vi "Cypher Lithography 2.0_Feng_MFP3D_Lucy.vi"(0 "Nodes on the line\n(  x      ,       y   )":dbl[][](array[numeric])=[[-5e-06, -5e-06], [5e-06, 5e-06]] min=-4.5e-05 max=4.5e-05 step=1e-09 format="%#_6pm", 1 "V":dbl[](array[numeric]), 2 "Litho Speed":dbl=5e-07 format="%#_6pm/s", 3 "Z SetPoint":dbl format="%#_6p", 4 "New nodes spacing":dbl=1e-06 format="%#_6pm", 5 "display wave":bool, 6 "Need interpolate new nodes?":bool, 7 "PID close":bool) -> ()   [LabVIEW 2016]
uses:
  Cypher XY LVDT Parameters_MFP3D_Lucy.vi
  <vilib>/Analysis/2dsp.llb/Resample (constant to constant,single -channel).vi
  <vilib>/Utility/file.llb/Write To Spreadsheet File (DBL).vi
  <vilib>/Analysis/NI_AALPro.lvlib
panel:
  out "size(s) 3":i32
  out "size(s) 2":i32[](array[numeric])
  out "size(s)":i32[](array[numeric])
  out "XY Graph":T1(graph)
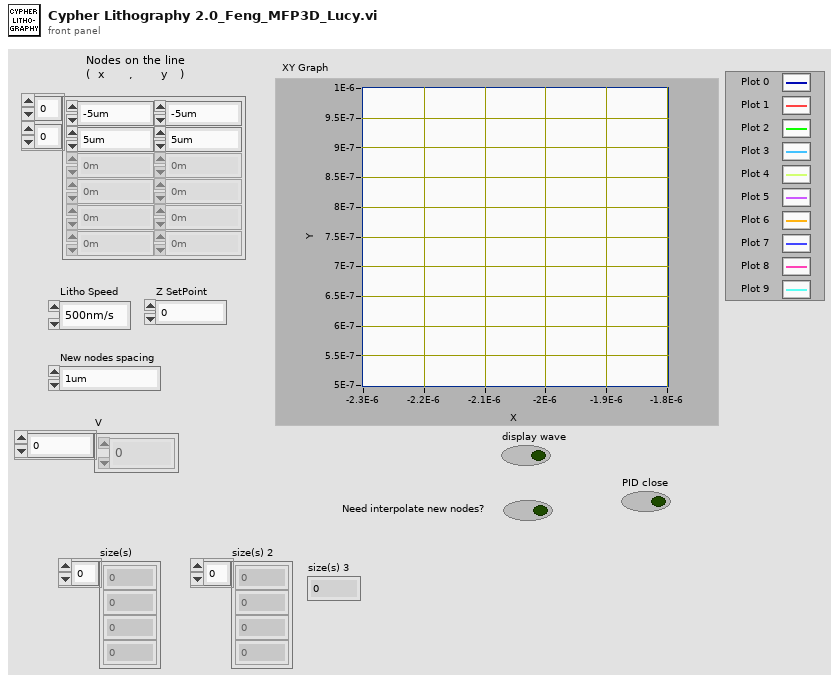
[diagram p1: front panel]
types:
  T1 = cluster{"Nodes on the line\n(  x      ,       y   )":dbl[], "Nodes on the line\n(  x      ,       y   )":dbl[]}[]
  T2 = cluster{"Interpolate result":dbl[], "Interpolate result":dbl[]}
  T3 = enum16{"open", "replace", "create", "open or create", "replace or create", "replace or create with confirmation"}
  T4 = cluster{"Nodes on the line\n(  x      ,       y   )":dbl[], "Nodes on the line\n(  x      ,       y   )":dbl[]}
  T5 = cluster{"Interpolate result":dbl[], "Interpolate result":dbl[]}[]
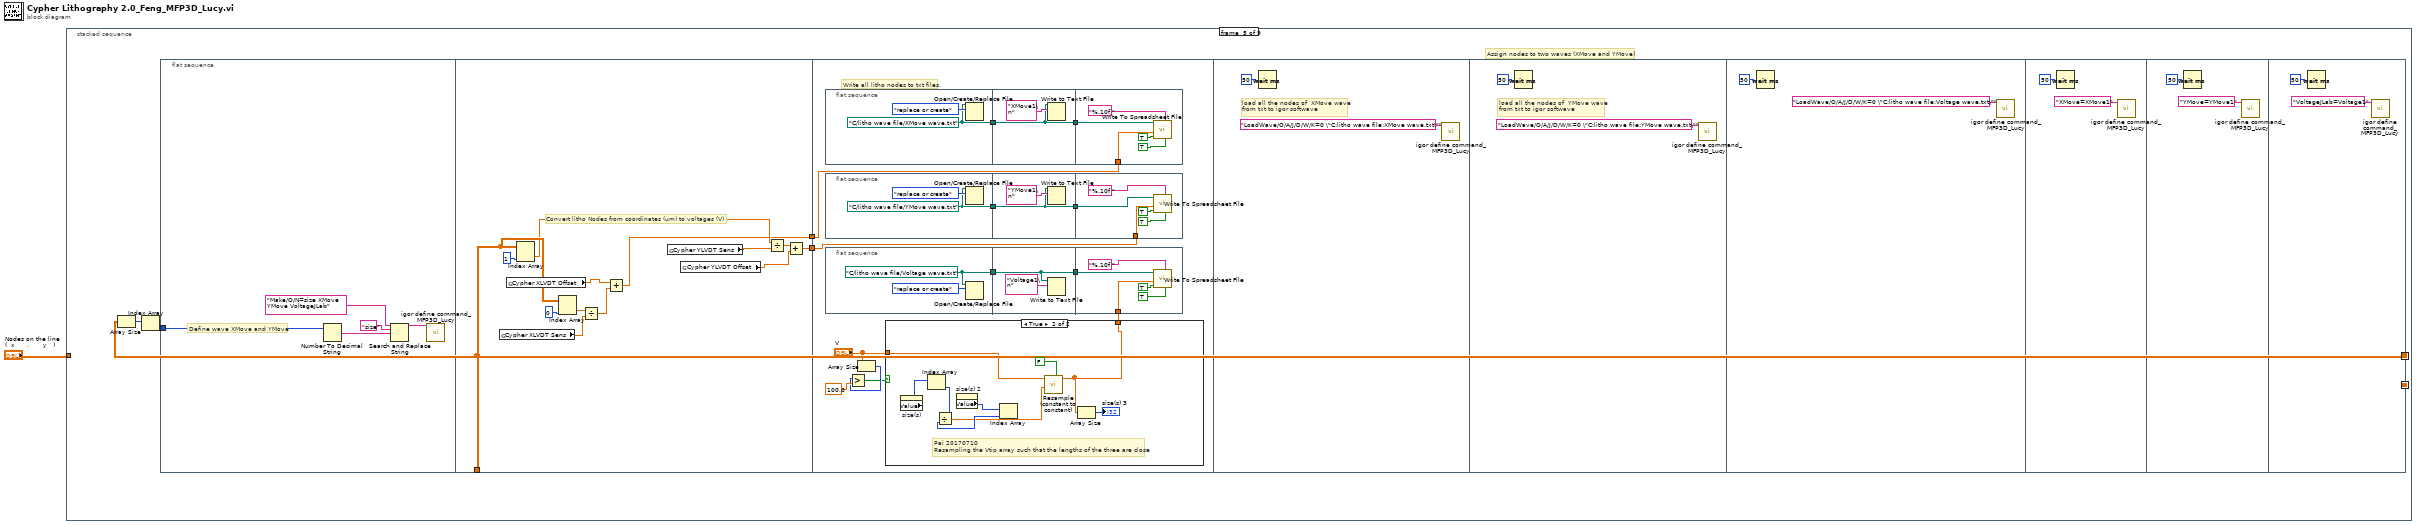
[diagram p0: block diagram]
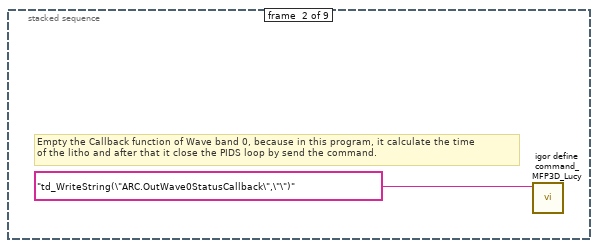
[diagram p3: hidden frame]
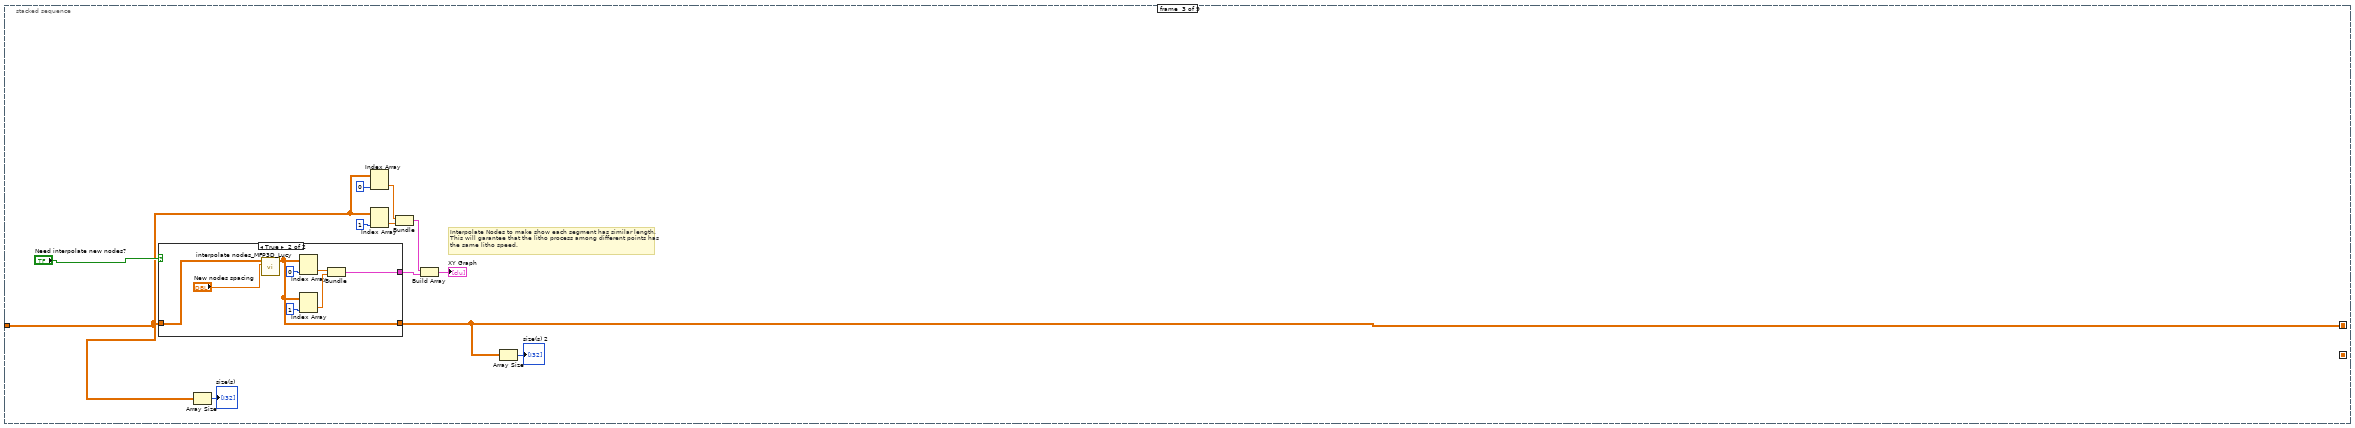
[diagram p4: hidden frame]
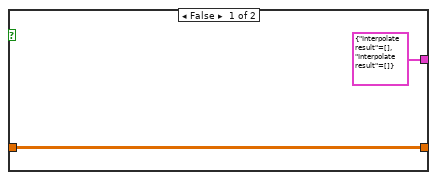
[diagram p5: hidden frame]
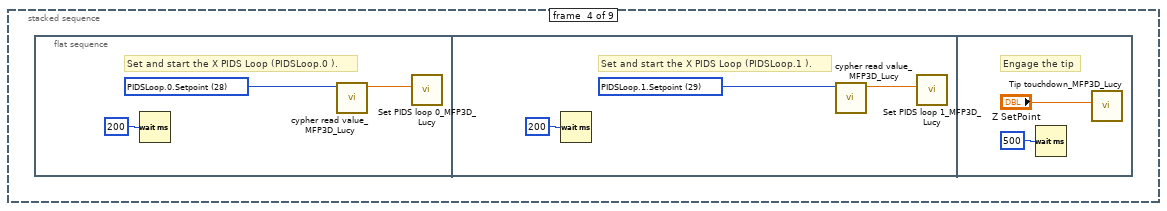
[diagram p6: hidden frame]
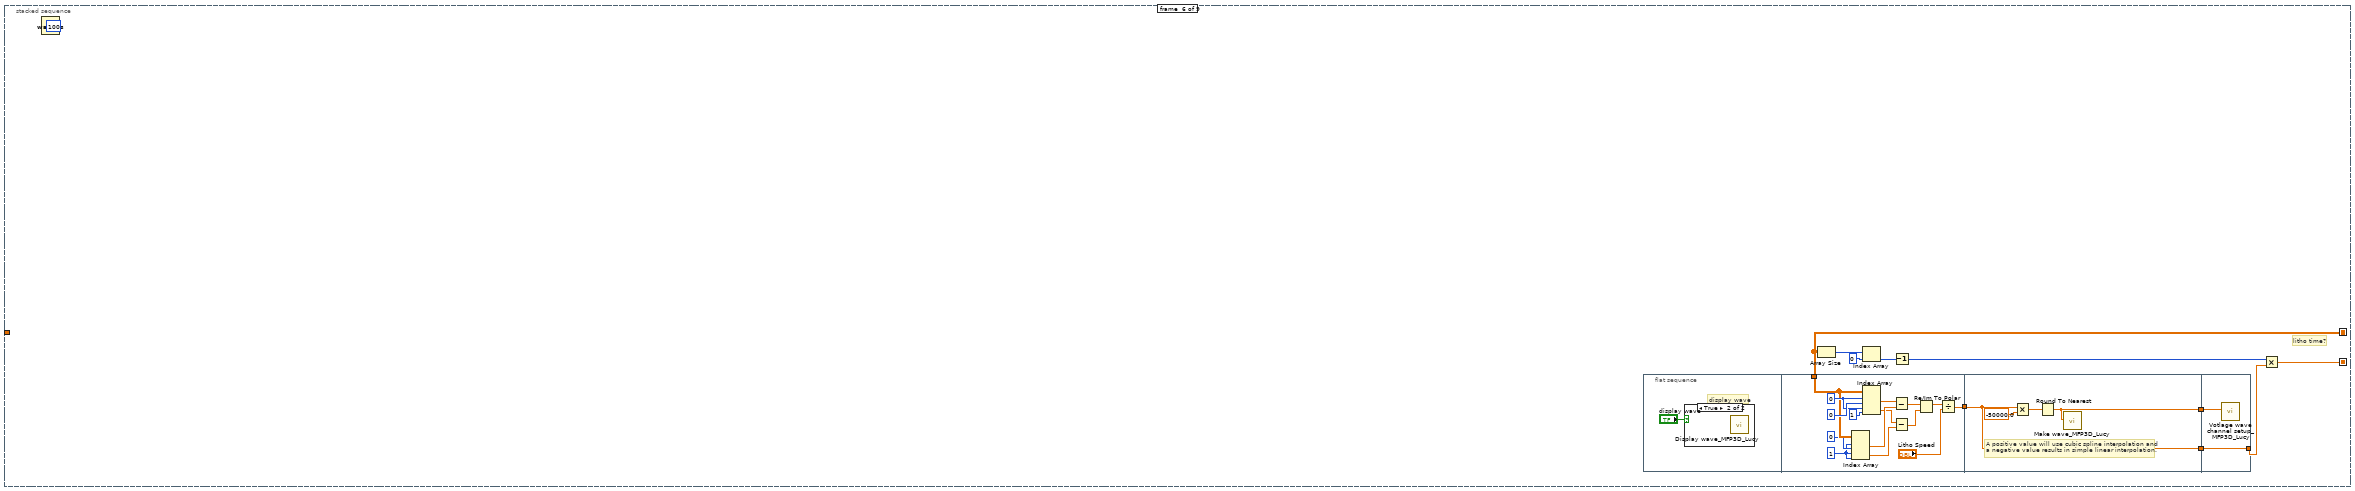
[diagram p8: hidden frame]
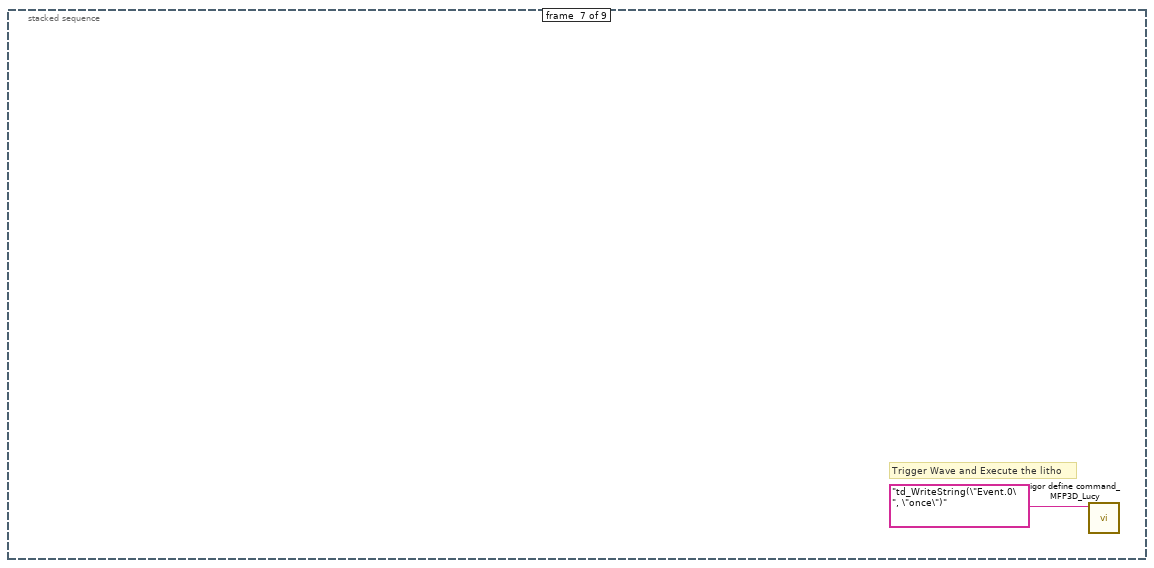
[diagram p10: hidden frame]
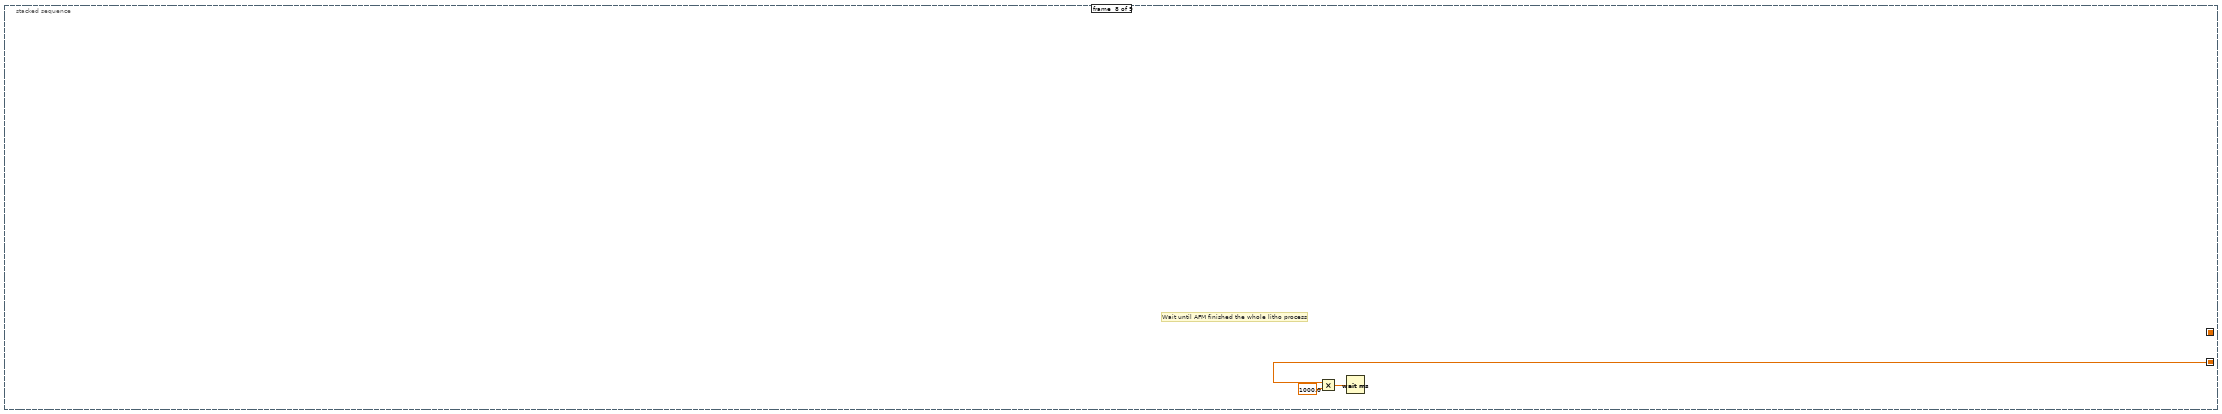
[diagram p11: hidden frame]
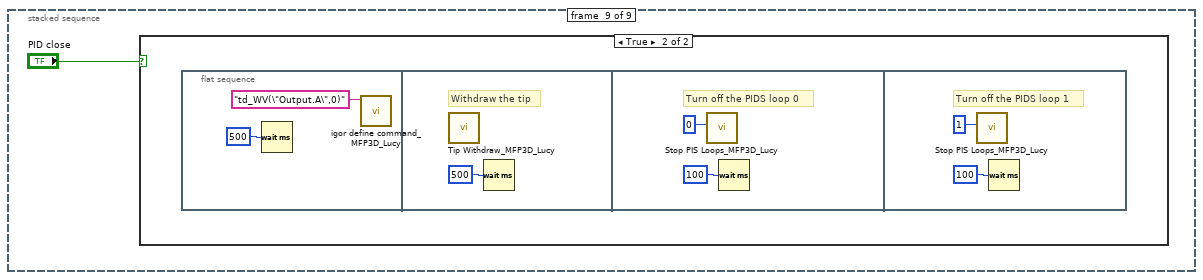
[diagram p12: hidden frame]
diagram:
  n1 = stacked-sequence {
    seq-local: [_ _ w3 _ _ _ _ _ _] -> [_ _ _ _ w34 w127 _ _ _]
    seq-local: [_ _ _ _ _ w123 _ _ _] -> [_ _ _ _ _ _ _ w154 _]
    tunnel: "Nodes on the line\n(  x      ,       y   )" -> [_ _ w6 _ _ _ _ _ _]
    frame #0 {
    }
    frame #1 {
      # "Empty the Callback function of Wave band 0, because in this program, it calculate the time \nof the litho and after that it close the PIDS loop by send the command."
      n2 = call "igor define command_MFP3D_Lucy.vi"("Command"="td_WriteString(\"ARC.OutWave0StatusCallback\",\"\")") -> ()  [unwired: 11 out]
    }
    frame #2 {
      # "Interpolate Nodes to make show each segment has similar length.\nThis will garantee that the litho process among different points has\nthe same litho speed."
      n3 = case shown="True" "Need interpolate new nodes?" {
        tunnel: w6 -> [w16 w17]
        tunnel: [T2 {"Interpolate result"=[], "Interpolate result"=[]} w20] -> w8
        tunnel: [w16 w19] -> w3
        frame False {
        }
        frame True {
          n4 = call "interpolate nodes_MFP3D_Lucy.vi"("Interpolate spacing"="New nodes spacing", "Nodes on the line\n(  x      ,       y   )"=w17) -> ("Interpolate result"=w19:dbl[][])  [unwired: 9 in]
          n5 = Index Array(array=w19, index (col)=0 ("disabled index (col)")) -> (element=w22:dbl[])  [unwired: 1 in]
          n6 = Index Array(array=w19, index (col)=1 ("disabled index (col)")) -> (element=w21:dbl[])  [unwired: 1 in]
          n7 = Bundle("Interpolate result"=w22, "Interpolate result"=w21) -> (w20:T2)  [unwired: 1 in]
        }
      }
      n8 = Array Size(array=w6) -> (size(s)=→"size(s)":i32[])
      n9 = Index Array(array=w6, index (col)=0 ("disabled index (col)")) -> (element=w13:dbl[])  [unwired: 1 in]
      n10 = Index Array(array=w6, index (col)=1 ("disabled index (col)")) -> (element=w11:dbl[])  [unwired: 1 in]
      n11 = Bundle("Nodes on the line\n(  x      ,       y   )"=w13, "Nodes on the line\n(  x      ,       y   )"=w11) -> (w10:T4)  [unwired: 1 in]
      n12 = Build Array(w10, w8) -> (→"XY Graph":T5)
      n13 = Array Size(array=w3) -> (size(s)=→"size(s) 2":i32[])
    }
    frame #3 {
      n14 = flat-sequence {
        frame #0 {
          w26 = u16 28 items=["XSensor", "YSensor", "ZSensor", "InA", "InB", "InFast", "In_Amplitude1", "In_Amplitude2", "In_Phase1", "In_Phase2", "PiezoX", "PiezoY", "PiezoZ", "OutA", "OutB", "OutC", "DDS_Frequency1", "DDS_Frequency2", "DDS_Amplitude1", "DDS_Amplitude2", "DDS_DCOffset", "Laser_Sum", "Laser_Difference", "Laser_Lateral", "XLVDT Sensitivity", "YLVDT Sensitivity", "XLVDT Offset", "YLVDT Offset", "PIDSLoop.0.Setpoint", "PIDSLoop.1.Setpoint"] ("Input")
          # "Set and start the X PIDS Loop (PIDSLoop.0 )."
          n15 = Wait (ms)(milliseconds to wait=u32 200) -> ()  [unwired: 1 out]
          n16 = call "cypher read value_MFP3D_Lucy.vi"("Input"=w26) -> ("Result"=w27:dbl)  [unwired: 10 in]
          n17 = call "Set PIDS loop 0_MFP3D_Lucy.vi"("X  Setpoint"=w27) -> ()  [unwired: 11 in]
        }
        frame #1 {
          w29 = u16 29 items=["XSensor", "YSensor", "ZSensor", "InA", "InB", "InFast", "In_Amplitude1", "In_Amplitude2", "In_Phase1", "In_Phase2", "PiezoX", "PiezoY", "PiezoZ", "OutA", "OutB", "OutC", "DDS_Frequency1", "DDS_Frequency2", "DDS_Amplitude1", "DDS_Amplitude2", "DDS_DCOffset", "Laser_Sum", "Laser_Difference", "Laser_Lateral", "XLVDT Sensitivity", "YLVDT Sensitivity", "XLVDT Offset", "YLVDT Offset", "PIDSLoop.0.Setpoint", "PIDSLoop.1.Setpoint"] ("Input")
          # "Set and start the X PIDS Loop (PIDSLoop.1 )."
          n18 = Wait (ms)(milliseconds to wait=u32 200) -> ()  [unwired: 1 out]
          n19 = call "cypher read value_MFP3D_Lucy.vi"("Input"=w29) -> ("Result"=w30:dbl)  [unwired: 10 in]
          n20 = call "Set PIDS loop 1_MFP3D_Lucy.vi"("Y Setpoint"=w30) -> ()  [unwired: 11 in]
        }
        frame #2 {
          # "Engage the tip"
          n21 = Wait (ms)(milliseconds to wait=u32 500) -> ()  [unwired: 1 out]
          n22 = call "Tip touchdown_MFP3D_Lucy.vi"("Z SetPoint"="Z SetPoint") -> ()  [unwired: 11 out]
        }
      }
    }
    frame #4 {
      # "Assign nodes to two waves (XMove and YMove)"
      n23 = Array Size(array=w34) -> (size(s)=w35:i32[])
      n24 = Index Array(array=w35) -> (element=w33:i32)  [unwired: 1 in]
      n25 = flat-sequence {
        tunnel: w33 -> [w38]
        tunnel: w34 -> [w52]
        tunnel: [w48] -> w37
        tunnel: [w47] -> w36
        tunnel: w37 -> [w64]
        tunnel: w36 -> [w63]
        frame #0 {
          # "Define wave XMove and YMove"
          n26 = Number To Decimal String(number=w38) -> (decimal integer string=w40:string)  [unwired: 1 in]
          n27 = Search and Replace String(input string="Make/O/N=size XMove YMove VoltageJLab", search string="size", replace string=w40) -> (result string=w39:string)  [unwired: 1 in, 7 out]
          n28 = call "igor define command_MFP3D_Lucy.vi"("Command"=w39) -> ()  [unwired: 11 out]
        }
        frame #1 {
          # "Convert litho Nodes from coordinates (um) to voltages (V)"
          n29 = global read "Cypher XY LVDT Parameters_MFP3D_Lucy.vi" "Cypher XLVDT Sens"() -> (w45:dbl)
          n30 = global read "Cypher XY LVDT Parameters_MFP3D_Lucy.vi" "Cypher XLVDT Offset"() -> (w46:dbl)
          n31 = Index Array(array=w52, index (col)=1 ("disabled index (col)")) -> (element=w49:dbl[])  [unwired: 1 in]
          n32 = Index Array(array=w52, index (col)=0 ("disabled index (col)")) -> (element=w50:dbl[])  [unwired: 1 in]
          n33 = Divide(x=w50, y=w45) -> (x/y=w54:dbl[])
          n34 = Add(x=w46, y=w54) -> (x+y=w47:dbl[])
          n35 = global read "Cypher XY LVDT Parameters_MFP3D_Lucy.vi" "Cypher YLVDT Sens"() -> (w44:dbl)
          n36 = global read "Cypher XY LVDT Parameters_MFP3D_Lucy.vi" "Cypher YLVDT Offset"() -> (w43:dbl)
          n37 = Divide(x=w49, y=w44) -> (x/y=w53:dbl[])
          n38 = Add(x=w53, y=w43) -> (x+y=w48:dbl[])
        }
        frame #2 {
          # "Write all litho nodes to txt files."
          n39 = flat-sequence {
            tunnel: [w97] -> w68
            tunnel: w68 -> [w99]
            tunnel: [w99] -> w67
            tunnel: w67 -> [w103]
            tunnel: w63 -> [w102]
            frame #0 {
              w97 = path "C:/litho wave file/XMove wave.txt" ("\"XMove wave\" file path")
              n40 = Open/Create/Replace File(file path (use dialog)=w97, operation (0:open)=T3."replace or create") -> ()  [unwired: 4 in, 3 out]
            }
            frame #1 {
              n41 = Write to Text File(file (use dialog)=w99, text="XMove1\n") -> ()  [unwired: 2 in, 3 out]
            }
            frame #2 {
              n42 = call-poly <vilib>:"Write To Spreadsheet File.vi"("transpose? (no:F)"=TRUE, "format (%.3f)"="%.10f ", "append to file? (new file:F)"=TRUE, "1D data"=w102, "file path (dialog if empty)"=w103) -> ()  [unwired: 3 in, 1 out]
            }
          }
          n43 = flat-sequence {
            tunnel: [w88] -> w66
            tunnel: w66 -> [w90]
            tunnel: [w90] -> w65
            tunnel: w65 -> [w94]
            tunnel: w64 -> [w93]
            frame #0 {
              w88 = path "C:/litho wave file/YMove wave.txt" ("\"YMove wave\" file path")
              n44 = Open/Create/Replace File(file path (use dialog)=w88, operation (0:open)=T3."replace or create") -> ()  [unwired: 4 in, 3 out]
            }
            frame #1 {
              n45 = Write to Text File(file (use dialog)=w90, text="YMove1\n") -> ()  [unwired: 2 in, 3 out]
            }
            frame #2 {
              n46 = call-poly <vilib>:"Write To Spreadsheet File.vi"("transpose? (no:F)"=TRUE, "format (%.3f)"="%.10f ", "append to file? (new file:F)"=TRUE, "1D data"=w93, "file path (dialog if empty)"=w94) -> ()  [unwired: 3 in, 1 out]
            }
          }
          n47 = flat-sequence {
            tunnel: [w79] -> w62
            tunnel: w62 -> [w81]
            tunnel: [w81] -> w61
            tunnel: w61 -> [w85]
            tunnel: w60 -> [w83]
            frame #0 {
              w79 = path "C:/litho wave file/Voltage wave.txt" ("file path (use dialog)")
              n48 = Open/Create/Replace File(file path (use dialog)=w79, operation (0:open)=T3."replace or create") -> ()  [unwired: 4 in, 3 out]
            }
            frame #1 {
              n49 = Write to Text File(file (use dialog)=w81, text="Voltage1\n") -> ()  [unwired: 2 in, 3 out]
            }
            frame #2 {
              n50 = call-poly <vilib>:"Write To Spreadsheet File.vi"("transpose? (no:F)"=TRUE, "format (%.3f)"="%.10f ", "append to file? (new file:F)"=TRUE, "1D data"=w83, "file path (dialog if empty)"=w85) -> ()  [unwired: 3 in, 1 out]
            }
          }
          n51 = Array Size(array="V") -> (size(s)=w57:i32)
          n52 = Greater?(x=w57, y=100.0) -> (0:w56:bool)
          n53 = case shown="True" w56 {
            tunnel: [w69 w78] -> w60
            tunnel: "V" -> [w69 w70]
            frame False {
            }
            frame True {
              # "Pai 20170710\nResampling the Vtip array such that the lengths of the three are close"
              n54 = property on="size(s)" class="Arr (strict)"() -> ("Value"=w75:i32[])  [unwired: 2 in, 2 out]
              n55 = Index Array(array=w75) -> (element=w74:i32)  [unwired: 1 in]
              n56 = property on="size(s) 2" class="Arr (strict)"() -> ("Value"=w73:i32[])  [unwired: 2 in, 2 out]
              n57 = Index Array(array=w73) -> (element=w72:i32)  [unwired: 1 in]
              n58 = Divide(x=w74, y=w72) -> (x/y=w71:dbl)
              n59 = call-poly <vilib>:"Resample (constant to constant).vi"("anti-aliasing?"=FALSE, "dt"=w71, "X"=w70) -> ("Y"=w78:dbl[])  [unwired: 6 in, 2 out]
              n60 = Array Size(array=w78) -> (size(s)=→"size(s) 3":i32)
            }
          }
        }
        frame #3 {
          # "load all the nodes of  XMove wave\nfrom txt to igor softwave"
          n61 = Wait (ms)(milliseconds to wait=u32 50) -> ()  [unwired: 1 out]
          n62 = call "igor define command_MFP3D_Lucy.vi"("Command"="LoadWave/O/A/J/D/W/K=0 \"C:litho wave file:XMove wave.txt\"") -> ()  [unwired: 11 out]
        }
        frame #4 {
          # "load all the nodes of  YMove wave\nfrom txt to igor softwave"
          n63 = Wait (ms)(milliseconds to wait=u32 50) -> ()  [unwired: 1 out]
          n64 = call "igor define command_MFP3D_Lucy.vi"("Command"="LoadWave/O/A/J/D/W/K=0 \"C:litho wave file:YMove wave.txt\"") -> ()  [unwired: 11 out]
        }
        frame #5 {
          n65 = Wait (ms)(milliseconds to wait=u32 50) -> ()  [unwired: 1 out]
          n66 = call "igor define command_MFP3D_Lucy.vi"("Command"="LoadWave/O/A/J/D/W/K=0 \"C:litho wave file:Voltage wave.txt\"") -> ()  [unwired: 11 out]
        }
        frame #6 {
          n67 = Wait (ms)(milliseconds to wait=u32 50) -> ()  [unwired: 1 out]
          n68 = call "igor define command_MFP3D_Lucy.vi"("Command"="XMove=XMove1") -> ()  [unwired: 11 out]
        }
        frame #7 {
          n69 = Wait (ms)(milliseconds to wait=u32 50) -> ()  [unwired: 1 out]
          n70 = call "igor define command_MFP3D_Lucy.vi"("Command"="YMove=YMove1") -> ()  [unwired: 11 out]
        }
        frame #8 {
          n71 = Wait (ms)(milliseconds to wait=u32 50) -> ()  [unwired: 1 out]
          n72 = call "igor define command_MFP3D_Lucy.vi"("Command"="VoltageJLab=Voltage1") -> ()  [unwired: 11 out]
        }
      }
    }
    frame #5 {
      # "litho time?"
      n73 = Wait (ms)(milliseconds to wait=u32 100) -> ()  [unwired: 1 out]
      n74 = flat-sequence {
        tunnel: w127 -> [w141]
        tunnel: [w130] -> w128
        tunnel: w128 -> [w146]
        tunnel: [w146] -> w119
        tunnel: [w145] -> w118
        tunnel: [w150] -> w124
        tunnel: w119 -> [w150]
        tunnel: w118 -> [w149]
        frame #0 {
          # "display wave"
          n75 = case shown="True" "display wave" {
            frame False {
            }
            frame True {
              n76 = call "Display wave_MFP3D_Lucy.vi"() -> ()  [unwired: 1 out]
            }
          }
        }
        frame #1 {
          w139 = 1 ("index (row)")
          w143 = 0 ("index (row)")
          n77 = Index Array(array=w141, index (row) #1=w139, index (col) #1=0 ("disabled index (col)"), index (row) #2=w139, index (col) #2=w139) -> (element #1=w137:dbl, element #2=w136:dbl)
          n78 = Index Array(array=w141, index (row) #1=w143, index (col) #1=0 ("disabled index (col)"), index (row) #2=w143, index (col) #2=1 ("disabled index (col)")) -> (element #1=w138:dbl, element #2=w135:dbl)
          n79 = Subtract(x=w138, y=w137) -> (x-y=w134:dbl)
          n80 = Subtract(x=w135, y=w136) -> (x-y=w133:dbl)
          n81 = Re/Im To Polar(2:w133, 3:w134) -> (1:w132:dbl)  [unwired: 1 out]
          n82 = Divide(x=w132, y="Litho Speed") -> (x/y=w130:dbl)
        }
        frame #2 {
          # "A positive value will use cubic spline interpolation and \na negative value results in simple linear interpolation."
          n83 = Multiply(x=w146, y=-50000.0) -> (x*y=w147:dbl)
          n84 = Round To Nearest(number=w147) -> (nearest integer value=w145:dbl)
          n85 = call "Make wave_MFP3D_Lucy.vi"("Totalpoints"=w145) -> ()  [unwired: 11 out]
        }
        frame #3 {
          n86 = call "Votlage wave channel setup_MFP3D_Lucy.vi"("Totalpoints"=w149) -> ()  [unwired: 11 in]
        }
      }
      n87 = Array Size(array=w127) -> (size(s)=w126:i32[])
      n88 = Index Array(array=w126, index=0) -> (element=w122:i32)
      n89 = Decrement(x=w122) -> (x-1=w121:i32)
      n90 = Multiply(x=w121, y=w124) -> (x*y=w123:dbl)
    }
    frame #6 {
      # "Trigger Wave and Execute the litho"
      n91 = call "igor define command_MFP3D_Lucy.vi"("Command"="td_WriteString(\"Event.0\", \"once\")") -> ()  [unwired: 11 out]
    }
    frame #7 {
      # "Wait until AFM finished the whole litho process"
      n92 = Multiply(x=w154, y=1000.0) -> (x*y=w152:dbl)
      n93 = Wait (ms)(milliseconds to wait=w152) -> ()  [unwired: 1 out]
    }
    frame #8 {
      n94 = case shown="True" "PID close" {
        frame False {
        }
        frame True {
          n95 = flat-sequence {
            frame #0 {
              n96 = Wait (ms)(milliseconds to wait=u32 500) -> ()  [unwired: 1 out]
              n97 = call "igor define command_MFP3D_Lucy.vi"("Command"="td_WV(\"Output.A\",0)") -> ()  [unwired: 11 out]
            }
            frame #1 {
              # "Withdraw the tip"
              n98 = call "Tip Withdraw_MFP3D_Lucy.vi"() -> ()  [unwired: 1 in]
              n99 = Wait (ms)(milliseconds to wait=u32 500) -> ()  [unwired: 1 out]
            }
            frame #2 {
              # "Turn off the PIDS loop 0"
              n100 = call "Stop PIS Loops_MFP3D_Lucy.vi"("PIS Loop Number (0-5)"=u32 0) -> ()  [unwired: 11 out]
              n101 = Wait (ms)(milliseconds to wait=u32 100) -> ()  [unwired: 1 out]
            }
            frame #3 {
              # "Turn off the PIDS loop 1"
              n102 = call "Stop PIS Loops_MFP3D_Lucy.vi"("PIS Loop Number (0-5)"=u32 1) -> ()  [unwired: 11 out]
              n103 = Wait (ms)(milliseconds to wait=u32 100) -> ()  [unwired: 1 out]
            }
          }
        }
      }
    }
  }
